vi "ExSubSetInitCam.vi"(0 "Camera Handle":u32, 1 "Exposure":dbl min=0.0 step=0.001 format="%.3f", 2 "Intensifier":bool, 3 "error in (no error)":errorcluster, 4 "Name":string) -> (5 "Handles Out":T1, 6 "error out":errorcluster)   [LabVIEW 2010]
panel:
  # "ExSubSetInitCam:\nThis sub vi initializes the camera."
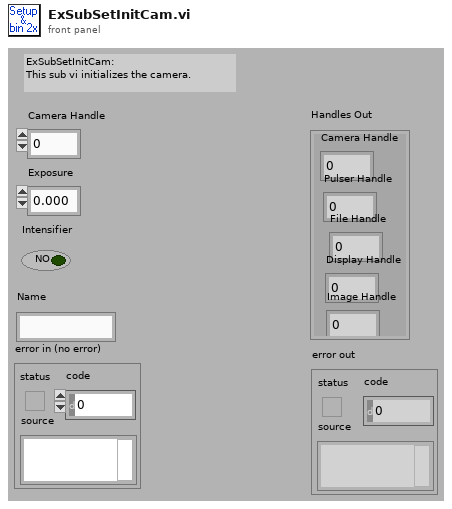
[diagram p1: front panel]
types:
  T1 = cluster{"Camera Handle":u32, "Pulser Handle":u32, "File Handle":u32, "Display Handle":u32, "Image Handle":u32}
  T2 = cluster{"acquire focus mode":u32, "Exposure":dbl, "Number of Images":u32, "Software accumulation":u32}
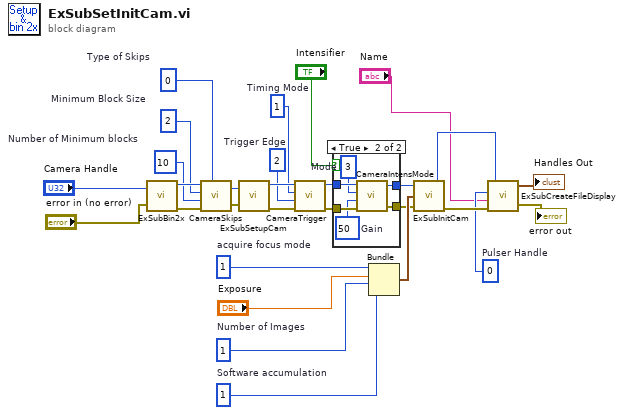
[diagram p0: block diagram]
diagram:
  w12 = u32 0  # Pulser Handle
  w13 = u32 1  # Timing Mode
  w14 = u32 2  # Trigger Edge
  w17 = u32 1  # acquire focus mode
  w16 = u32 1  # Number of Images
  w15 = u32 1  # Software accumulation
  w18 = u32 0  # Type of Skips
  w19 = u32 2  # Minimum Block Size
  w20 = u32 10  # Number of Minimum blocks
  n1 = call "ExSubBin2x.vi"("error in (no error)"="error in (no error)", "Camera Handle"="Camera Handle") -> ("error out"=w21:errorcluster, "Camera Handle"=w22:u32)
  n2 = call <userlib>:"CameraSkips.vi"("Camera Handle"=w22, "Minimum Block Size"=w19, "Number of Minimum blocks"=w20, "error in"=w21, "Type of Skips"=w18) -> ("Camera Handle"=w24:u32, "error out"=w23:errorcluster)
  n3 = call "ExSubSetupCam.vi"("error in (no error)"=w23, "Camera Handle"=w24) -> ("error out"=w25:errorcluster, "Camera Handle"=w26:u32)
  n4 = call <userlib>:"CameraTrigger.vi"("error in"=w25, "Trigger Edge"=w14, "Timing Mode"=w13, "Camera Handle"=w26) -> ("error out"=w9:errorcluster, "Camera Handle"=w11:u32)
  n5 = case shown="True" "Intensifier" {
    tunnel: w11 -> [w31 w37]
    tunnel: [w31 w36] -> w10
    tunnel: w9 -> [w30 w35]
    tunnel: [w30 w34] -> w8
    frame False {
    }
    frame True {
      w32 = u32 50  # Gain
      w33 = u32 3  # Mode
      n6 = call <userlib>:"CameraIntensMode.vi"("error in"=w35, "Intensifier Gain"=w32, "Mode"=w33, "Camera Handle"=w37) -> ("error out"=w34:errorcluster, "Camera Handle"=w36:u32)
    }
  }
  n7 = Bundle("acquire focus mode"=w17, "Exposure"="Exposure", "Number of Images"=w16, "Software accumulation"=w15) -> (w28:T2)  [unwired: 1 in]
  n8 = call "ExSubInitCam.vi"("error in (no error)"=w8, "Camera Information"=w28, "Camera Handle"=w10) -> ("error out"=w27:errorcluster, "Camera Handle"=w3:u32)
  n9 = call "ExSubCreateFileDisplay.vi"("error in (no error)"=w27, "File and Display Name"="Name", "Pulser Handle"=w12, "Camera Handle"=w3) -> ("error out"=→"error out":errorcluster, "Handles Out"=→"Handles Out":T1)
